vi "main Pos Processamento.vi"(1 "path":path) -> ()   [LabVIEW 2019]
panel:
  out "filenames":string[](array[string])
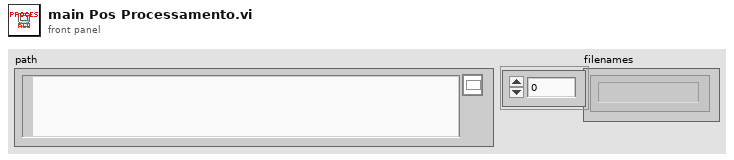
[diagram p1: front panel]
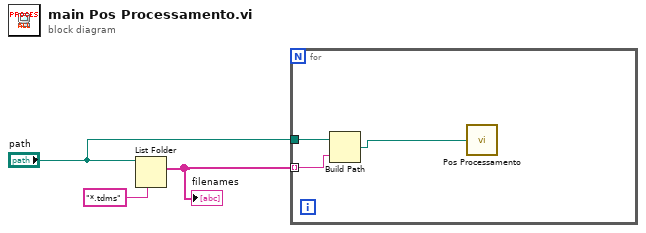
[diagram p0: block diagram]
diagram:
  n1 = List Folder(path="path", pattern="*.tdms") -> (filenames=w3:string[])  [unwired: 2 in, 3 out]
  "filenames" <- w3
  n2 = for {
    tunnel: w3 -> [w6] mode=indexing
    tunnel: "path" -> [w5]
    n3 = Build Path(base path=w5, name or relative path=w6) -> (appended path=w4:path)
    n4 = call "Pos Processamento.vi"("file path"=w4) -> ()  [unwired: 1 in]
  }
